vi "Get or Add Row.vi"(8 "error in":errorcluster, 10 "Row Index":i32, 11 "Worksheet in":refnum<k24>) -> (0 "error out":errorcluster, 2 "Row":refnum<k24>, 3 "Worksheet out":refnum<k24>)   [LabVIEW 2019, in "Open Xml.lvlib"]
uses:
  Open Xml.lvlib
  D:/git/Open-Xml-LabVIEW/Source/DocumentFormat.OpenXml.dll
  DocumentFormat.OpenXml.dll
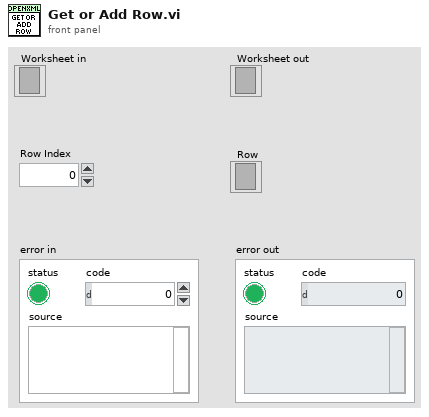
[diagram p1: front panel]
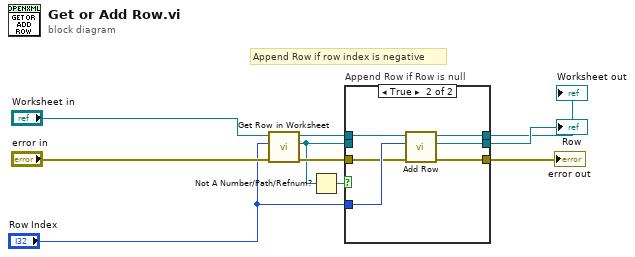
[diagram p0: block diagram]
diagram:
  # "Append Row if row index is negative"
  n1 = call "Get Row in Worksheet.vi"("error in"="error in", "RowIndex"="Row Index", "Worksheet in"="Worksheet in") -> ("error out"=w7:errorcluster, "Row out"=w4:refnum<k24>, "Worksheet out"=w6:refnum<k24>)  [unwired: 6 in]
  n2 = Not A Number/Path/Refnum?(number/path/refnum=w4) -> (NaN/Path/Refnum?=w9:bool)
  n3 = case "Append Row if Row is null" shown="True" w9 {
    tunnel: "Row Index" -> [_ w19]
    tunnel: w7 -> [w13 w18]
    tunnel: w6 -> [w11 w17]
    tunnel: [w13 w16] -> w2
    tunnel: [w12 w15] -> w5
    tunnel: w4 -> [w12 _]
    tunnel: [w11 w14] -> w1
    frame False {
    }
    frame True {
      n4 = call "Add Row.vi"("error in"=w18, "RowIndex"=w19, "Worksheet in"=w17) -> ("error out"=w16:errorcluster, "Row"=w15:refnum<k24>, "Worksheet out"=w14:refnum<k24>)  [unwired: 6 in]
    }
  }
  "error out" <- w2
  "Row" <- w5
  "Worksheet out" <- w1
